vi "DSF.Engine.Plugin.Response.Receive.vi"(8 "error in (no error)":errorcluster, 9 "timeout in ms (0)":i32 format="%d ms", 11 "Plugin in":refnum<class "DSF.Engine.Plugin.lvclass">) -> (0 "error out":errorcluster, 1 "timed out?":bool, 2 "response":T1, 3 "Plugin out":refnum<class "DSF.Engine.Plugin.lvclass">)   [LabVIEW 2017, in "DSF.Engine.lvlib" / "DSF.Engine.Plugin.lvclass"]
uses:
  DSF.Engine.Plugin.lvclass
  Interface/DSF.Engine.Interface.Plugin.Response Data.ctl
  Interface/DSF.Engine.Interface.Plugin.Response.ctl
  Interface/DSF.Engine.Interface.Plugin.Response Parameters.ctl
  DSF.Engine.Plugin.lvclass/DSF.Engine.Plugin.ctl
  Interface/DSF.Engine.Interface.Plugin.Read.Response.vi
  Interface/DSF.Engine.Interface.Plugin.lvclass
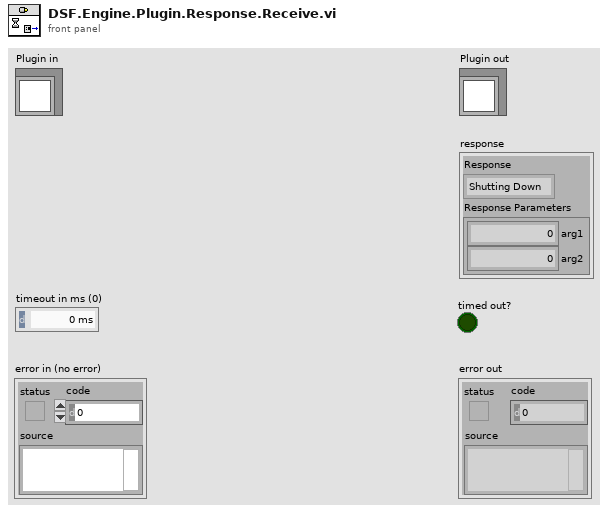
[diagram p1: front panel]
types:
  T1 = typedef "DSF.Engine.lvlib/DSF.Engine.Interface.Plugin.lvclass/DSF.Engine.Interface.Plugin.Response Data.ctl" = cluster{"Response":T2, "Response Parameters":T3}
  T2 = typedef "DSF.Engine.lvlib/DSF.Engine.Interface.Plugin.lvclass/DSF.Engine.Interface.Plugin.Response.ctl" = enum8{"Shutting Down"}
  T3 = typedef "DSF.Engine.lvlib/DSF.Engine.Interface.Plugin.lvclass/DSF.Engine.Interface.Plugin.Response Parameters.ctl" = cluster{"arg1":u64, "arg2":u64}
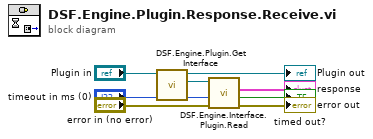
[diagram p0: block diagram]
diagram:
  n1 = call "DSF.Engine.Plugin.Get Interface.vi"("Plugin in"="Plugin in") -> ("Interface"=w7:refnum<class "DSF.Engine.Interface.Plugin.lvclass">, "Plugin out"=→"Plugin out":refnum<class "DSF.Engine.Plugin.lvclass">)  [unwired: 9 in]
  n2 = call-poly "DSF.Engine.Interface.Plugin.Read.vi"("error in (no error)"="error in (no error)", "timeout in ms (0)"="timeout in ms (0)", "Plugin Interface in"=w7) -> ("error out"=→"error out":errorcluster, "empty?"=→"timed out?":bool, "response"=→"response":T1)  [unwired: 4 in, 2 out]
